vi "Colour_Uncolour_List Item.vi"(7 "Enum":T1(ring), 8 "Error In":errorcluster, 10 "Index":i32, 11 "LstBox Refnum":refnum<vi>) -> (0 "Error Out":errorcluster)   [LabVIEW 2012]
doc: "SciScan 1.2 160622\nThsi VI changes the appearance of the specified list item to give the appearance of Selected and Deselected item."
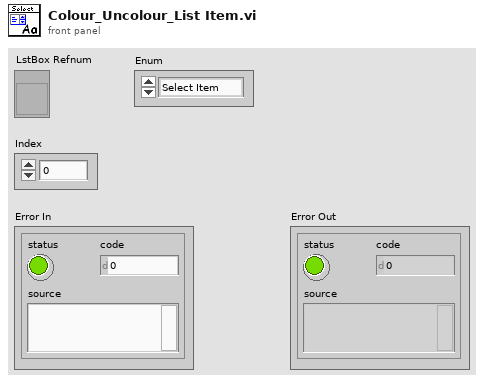
[diagram p1: front panel]
types:
  T1 = enum16{"Select Item", "Deselect Item", "Select All", "Deselect All"}
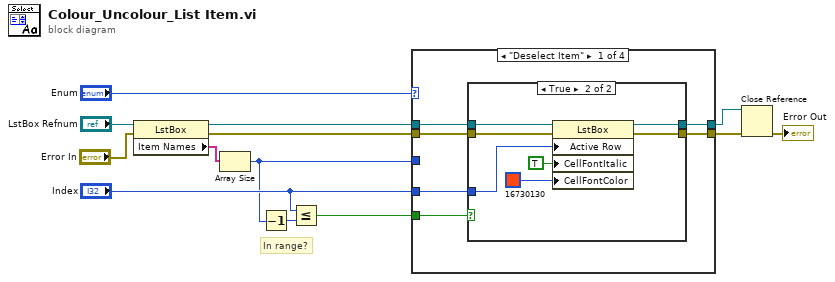
[diagram p0: block diagram]
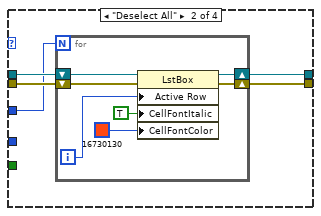
[diagram p3: hidden frame]
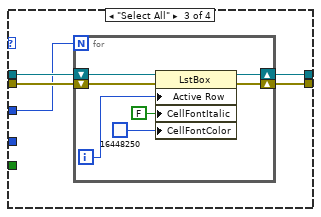
[diagram p4: hidden frame]
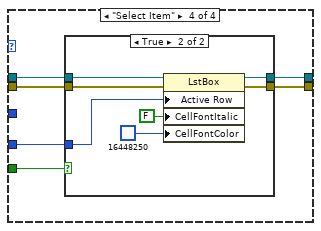
[diagram p5: hidden frame]
diagram:
  # "In range?"
  n1 = property class="LstBox"(reference="LstBox Refnum", error in="Error In") -> (reference out=w10:refnum<vi>, error out=w5:errorcluster, "Item Names"=w12:string[])
  n2 = Array Size(array=w12) -> (size(s)=w2:i32)
  n3 = Decrement(x=w2) -> (x-1=w9:i32)
  n4 = Less Or Equal?(x="Index", y=w9) -> (x <= y?=w8:bool)
  n5 = case shown="\"Deselect Item\"" "Enum" {
    tunnel: w10 -> [w19 w33 w45 w58]
    tunnel: w8 -> [w18 _ _ w57]
    tunnel: "Index" -> [w17 _ _ w56]
    tunnel: w5 -> [w16 w32 w44 w55]
    tunnel: [w15 w31 w43 w54] -> w1
    tunnel: [w14 w30 w42 w53] -> w3
    tunnel: w2 -> [_ w29 w41 _]
    frame "Deselect Item" {
      n6 = case shown="True" w18 {
        tunnel: w19 -> [w20 w28]
        tunnel: w17 -> [_ w27]
        tunnel: w16 -> [w21 w26]
        tunnel: [w21 w24] -> w15
        tunnel: [w20 w23] -> w14
        frame False {
        }
        frame True {
          n7 = property class="LstBox"(reference=w28, error in=w26, "Active Row"=w27, "CellFontItalic"=TRUE ("Active Row:Cell Font:Italic"), "CellFontColor"=u32 16730130) -> (reference out=w23:refnum<vi>, error out=w24:errorcluster)
        }
      }
    }
    frame "Deselect All" {
      n8 = for {
        N: w29 -> [_]
        shift-right: [w38] -> w31
        shift-left: w32 -> [w39]
        shift-right: [w37] -> w30
        shift-left: w33 -> [w40]
        i -> [w34]
        n9 = property class="LstBox"(reference=w40, error in=w39, "Active Row"=w34, "CellFontItalic"=TRUE ("Active Row:Cell Font:Italic"), "CellFontColor"=u32 16730130) -> (reference out=w37:refnum<vi>, error out=w38:errorcluster)
      }
    }
    frame "Select All" {
      n10 = for {
        N: w41 -> [_]
        shift-right: [w50] -> w43
        shift-left: w44 -> [w51]
        shift-right: [w49] -> w42
        shift-left: w45 -> [w52]
        i -> [w46]
        n11 = property class="LstBox"(reference=w52, error in=w51, "Active Row"=w46, "CellFontItalic"=FALSE ("Active Row:Cell Font:Italic"), "CellFontColor"=u32 16448250) -> (reference out=w49:refnum<vi>, error out=w50:errorcluster)
      }
    }
    frame "Select Item" {
      n12 = case shown="True" w57 {
        tunnel: w58 -> [w59 w67]
        tunnel: w56 -> [_ w66]
        tunnel: w55 -> [w60 w65]
        tunnel: [w60 w62] -> w54
        tunnel: [w59 w61] -> w53
        frame False {
        }
        frame True {
          n13 = property class="LstBox"(reference=w67, error in=w65, "Active Row"=w66, "CellFontItalic"=FALSE ("Active Row:Cell Font:Italic"), "CellFontColor"=u32 16448250) -> (reference out=w61:refnum<vi>, error out=w62:errorcluster)
        }
      }
    }
  }
  n14 = Close Reference(reference=w3, error in (no error)=w1) -> (error out=→"Error Out":errorcluster)
